vi "Read Incoming Bytes.vi"(8 "error in (no error)":errorcluster, 9 "timeout (1000 ms)":i32=1000, 10 "bytes to read (100)":i32=100, 11 "TCPConnection in":refnum<class "LocalQueueConnection.lvclass">) -> (0 "error out":errorcluster, 1 "timed out":bool, 2 "Bytes":u8[](array[numeric]) format="%08b", 3 "TCPConnection out":refnum<class "LocalQueueConnection.lvclass">, 4 "connected":bool)   [LabVIEW 2013, in "MQTT_Queue.lvlib" / "LocalQueueConnection.lvclass"]
uses:
  LocalQueueConnection.lvclass
  LocalQueueConnection.lvclass/LocalQueueConnection.ctl
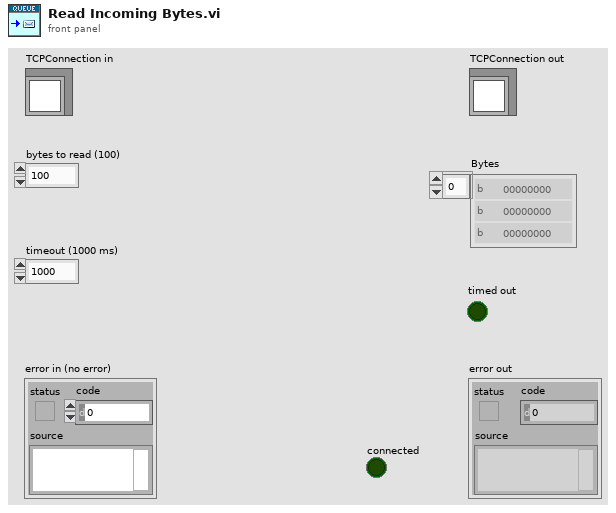
[diagram p1: front panel]
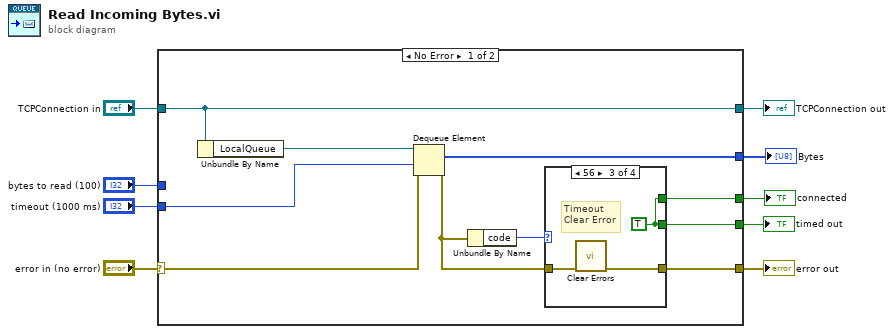
[diagram p0: block diagram]
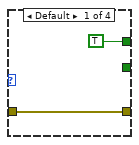
[diagram p2: hidden frame]
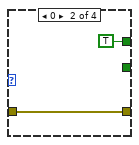
[diagram p3: hidden frame]
diagram:
  n1 = case shown="No Error" "error in (no error)" {
    selector: "error in (no error)" -> [w13 w29]
    tunnel: [w16 w29] -> w8
    tunnel: [w17 w28] -> w6
    tunnel: "TCPConnection in" -> [w17 w28]
    tunnel: [w12 _] -> w5
    tunnel: "bytes to read (100)" -> [_ _]
    tunnel: "timeout (1000 ms)" -> [w11 _]
    tunnel: [w18 _] -> w2
    tunnel: [w15 _] -> w1
    frame No Error {
      n2 = Unbundle By Name(w17) -> ("LocalQueue"=w14:refnum<queue>)
      n3 = Dequeue Element(queue=w14, timeout in ms (-1)=w11, error in (no error)=w13) -> (element=w12:u8[], error out=w10:errorcluster)  [unwired: 2 out]
      n4 = Unbundle By Name(w10) -> ("code"=w19:i32)
      n5 = case shown="56" w19 {
        tunnel: [w21 w23 w26 w27] -> w16
        tunnel: w10 -> [w21 w23 w25 w27]
        tunnel: [_ _ w24 _] -> w18
        tunnel: [TRUE TRUE w24 _] -> w15
        frame Default {
        }
        frame 0 {
        }
        frame 56 {
          w24 = TRUE
          # "Timeout\nClear Error"
          n6 = call <vilib>:"Clear Errors.vi"("error in (no error)"=w25) -> ("error out"=w26:errorcluster)  [unwired: 6 in]
        }
        frame 1 {
          # "Disconnection\nby peer"
        }
      }
    }
    frame Error {
    }
  }
  "error out" <- w8
  "TCPConnection out" <- w6
  "Bytes" <- w5
  "timed out" <- w2
  "connected" <- w1
